vi "01_MatchPattern.vi"(11 "String":string) -> (3 "count":i32)   [LabVIEW 2020, in "client.lvclass"]
uses:
  client.lvclass
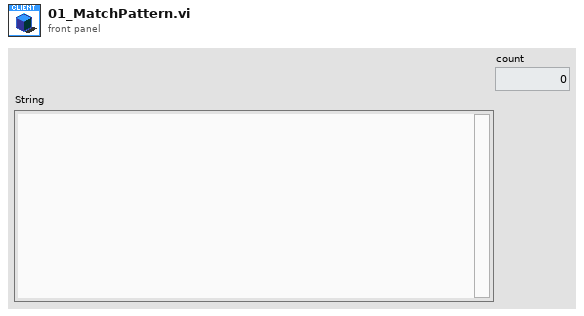
[diagram p1: front panel]
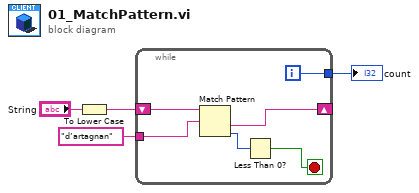
[diagram p0: block diagram]
diagram:
  n1 = To Lower Case(string="String") -> (all lower case string=w3:string)
  n2 = while {
    shift-right: [w9] -> _
    shift-left: w3 -> [w10]
    tunnel: "d’artagnan" -> [w8]
    tunnel: [w5] -> w1
    i -> [w5]
    stop <- w6 stop-if-true
    n3 = Match Pattern(string=w10, regular expression=w8) -> (after substring=w9:string, offset past match=w7:i32)  [unwired: 1 in, 2 out]
    n4 = Less Than 0?(x=w7) -> (x < 0?=w6:bool)
  }
  "count" <- w1
